vi "remove preceeding spaces.vi"(1 "Raw String":string) -> (0 "Edited String":string)   [LabVIEW 2021]
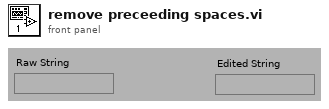
[diagram p1: front panel]
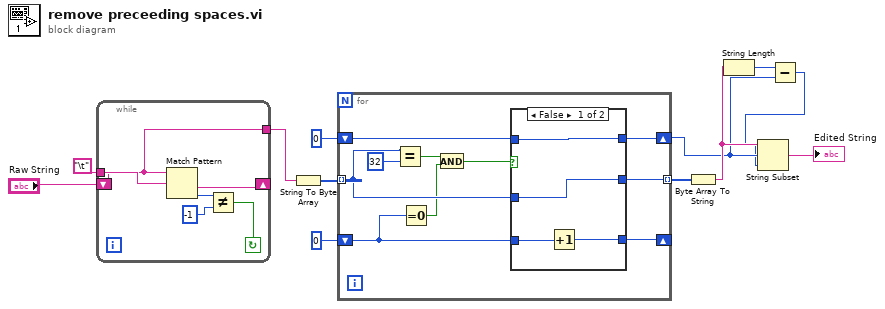
[diagram p0: block diagram]
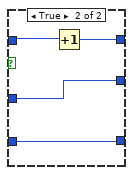
[diagram p2: hidden frame]
diagram:
  n1 = while {
    tunnel: [w13] -> w11
    tunnel: "\t" -> [w14]
    shift-left: "Raw String" -> [w13]
    shift-right: [w18] -> _
    stop <- w15 continue-if-true
    n2 = Match Pattern(string=w13, regular expression=w14) -> (after substring=w18:string, offset past match=w17:i32)  [unwired: 1 in, 2 out]
    n3 = Not Equal?(x=w17, y=-1) -> (x != y?=w15:bool)
  }
  n4 = String To Byte Array(string=w11) -> (unsigned byte array=w10:u8[])
  n5 = for {
    tunnel: w10 -> [w24] mode=indexing
    shift-right: [w26] -> _
    shift-left: u8 0 -> [w25]
    shift-right: [w23] -> w4
    shift-left: u8 0 -> [w22]
    tunnel: [w21] -> w7 mode=indexing
    n6 = Equal?(x=w24, y=u8 32) -> (x = y?=w27:bool)
    n7 = Equal To 0?(x=w25) -> (x = 0?=w19:bool)
    n8 = And(x=w27, y=w19) -> (x .and. y?=w20:bool)
    n9 = case shown="False" w20 {
      tunnel: w25 -> [w32 w33]
      tunnel: [w31 w33] -> w26
      tunnel: w24 -> [w30 w34]
      tunnel: [w30 w34] -> w21
      tunnel: [w29 w35] -> w23
      tunnel: w22 -> [w29 w36]
      frame False {
        n10 = Increment(x=w32) -> (x+1=w31:u8)
      }
      frame True {
        n11 = Increment(x=w36) -> (x+1=w35:u8)
      }
    }
  }
  n12 = Byte Array To String(unsigned byte array=w7) -> (string=w6:string)
  n13 = String Length(string=w6) -> (length=w5:i32)
  n14 = Subtract(x=w5, y=w4) -> (x-y=w3:i32)
  n15 = String Subset(string=w6, offset (0)=w4, length (rest)=w3) -> (substring=→"Edited String":string)
